vi "SaveSNP.vi"(6 "FileName":string, 7 "Ports":i32[](array[numeric])=[1], 8 "error in (no error)":errorcluster {"code" format="%.0x"}, 10 "Measurement":string, 11 "instrument handle":refnum<k15>) -> (0 "error out":errorcluster {"code" format="%.0x"}, 3 "instrument handle out":refnum<k15>)   [LabVIEW 2014, in "Agilent NA.lvlib"]
doc: "Save the SNP for this measurement"
uses:
  Agilent NA.lvlib
  AgNA.dll
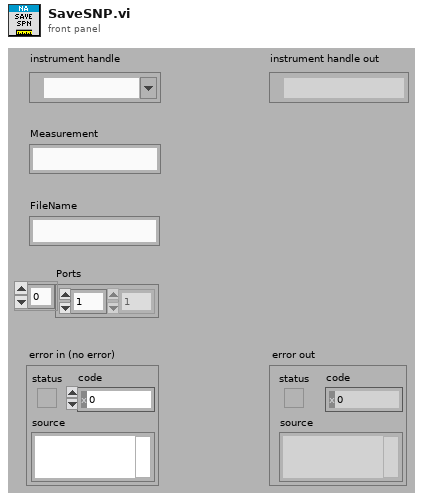
[diagram p1: front panel]
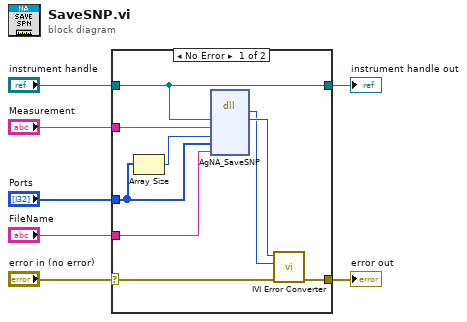
[diagram p0: block diagram]
diagram:
  n1 = case shown="No Error" "error in (no error)" {
    selector: "error in (no error)" -> [w14 w18]
    tunnel: [w13 w18] -> w7
    tunnel: "Measurement" -> [w12 _]
    tunnel: "Ports" -> [w8 _]
    tunnel: "FileName" -> [w11 _]
    tunnel: [w10 w17] -> w2
    tunnel: "instrument handle" -> [w10 w17]
    frame No Error {
      n2 = Array Size(array=w8) -> (size(s)=w9:i32)
      n3 = dll-call lib="AgNA**.dll" fn="AgNA_SaveSNP"("Vi"=w10, "Measurement"=w12, "PortsBufferSize"=w9, "Ports"=w8, "FileName"=w11) -> (w15:i32, "Vi"=w16:u32)  [unwired: 7 in, 2 out]
      n4 = call "IVI Error Converter.vi"("error in (no error)"=w14, "IVI error code (0)"=w15, "instrument handle"=w16) -> ("error out"=w13:errorcluster)  [unwired: 7 in, 1 out]
    }
    frame Error {
    }
  }
  "error out" <- w7
  "instrument handle out" <- w2
